vi "Init Sound Buffer.vi"(5 "Number of Samples":i32, 7 "Rx IQ Sampling\nRate [s/sec]":dbl, 11 "sound format":T1={"sample rate (S/s)"=44100.0, "number of channels"=2, "bits per sample"=16}) -> (0 "Samples/ch":i32, 1 "Allocated Waveform":waveform(dbl), 2 "dt":dbl)   [LabVIEW 2013]
uses:
  <vilib>/sound2/lvsound2.llb/Sound Data Format.ctl
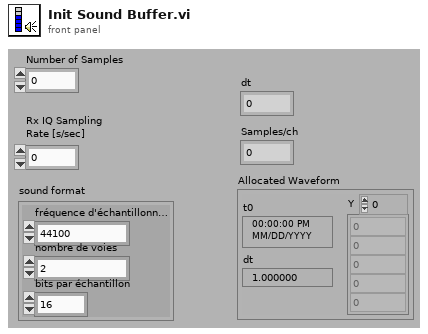
[diagram p1: front panel]
types:
  T1 = typedef "Sound Data Format.ctl" = cluster{"sample rate (S/s)":dbl, "number of channels":i32, "bits per sample":i32}
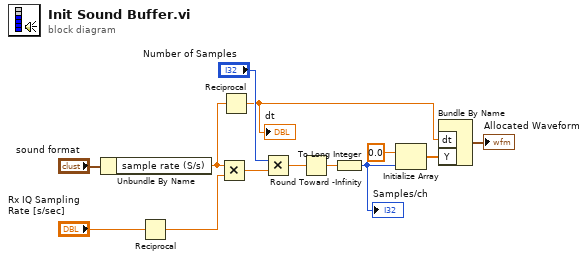
[diagram p0: block diagram]
diagram:
  n1 = Unbundle By Name("sound format") -> ("sample rate (S/s)"=w10:dbl)
  n2 = Reciprocal(x="Rx IQ Sampling\nRate [s/sec]") -> (1/x=w8:dbl)
  n3 = Multiply(x=w10, y=w8) -> (x*y=w6:dbl)
  n4 = Reciprocal(x=w10) -> (1/x=w9:dbl)
  "dt" <- w9
  n5 = Multiply(x="Number of Samples", y=w6) -> (x*y=w4:dbl)
  n6 = Round Toward -Infinity(1:w4) -> (0:w5:dbl)
  n7 = To Long Integer(number=w5) -> (32bit integer=w1:i32)
  "Samples/ch" <- w1
  n8 = Initialize Array(0.0 ("element"), w1) -> (w7:dbl[])
  n9 = Bundle By Name("dt"=w9, "Y"=w7) -> (→"Allocated Waveform":waveform(dbl))  [unwired: 1 in]
